vi "read_data_package.vi"(8 "error in (no error)":errorcluster, 11 "OXY_SCPI Reseource In":refnum<visa-resource-name>) -> (0 "error out":errorcluster, 1 "Complete Raw data":string, 2 "Package without Header":string, 3 "OXY_SCPI Reseource Out":refnum<visa-resource-name>)   [LabVIEW 2020, in "OXYGEN_Datastream.lvlib"]
uses:
  OXYGEN_Datastream.lvlib
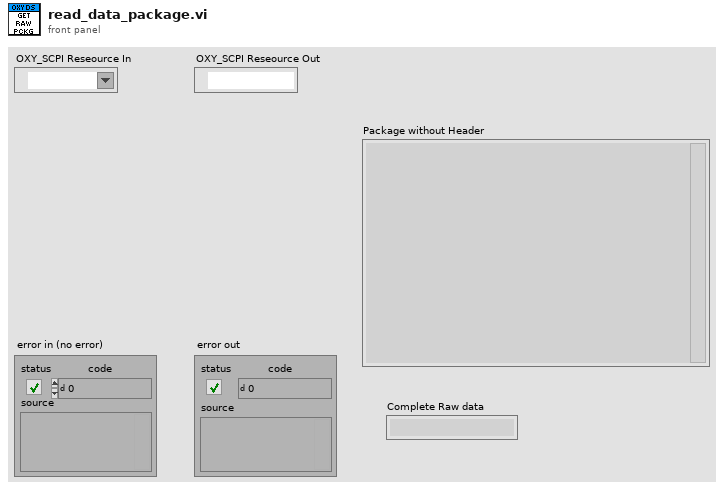
[diagram p1: front panel]
types:
  T1 = enum16{"big-endian, network order", "native, host order", "little-endian"}
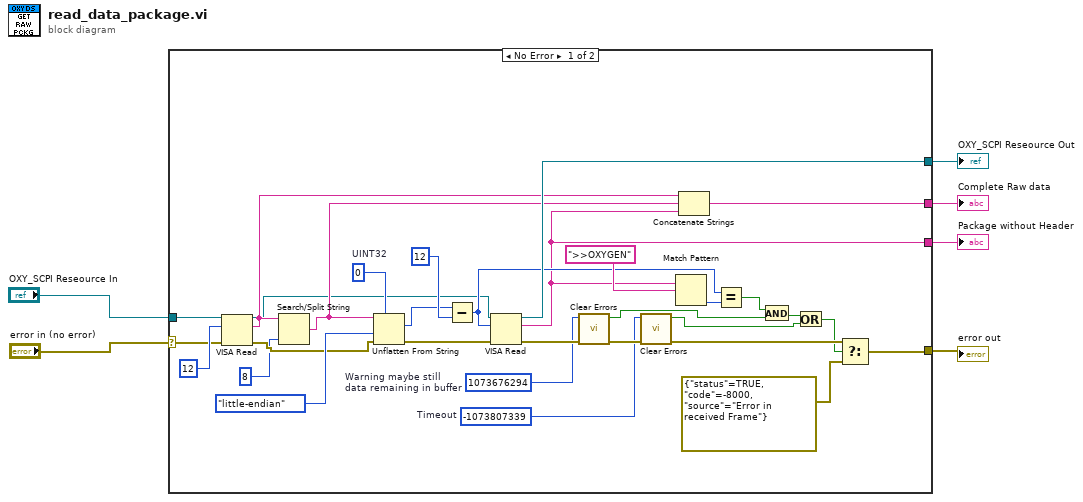
[diagram p0: block diagram]
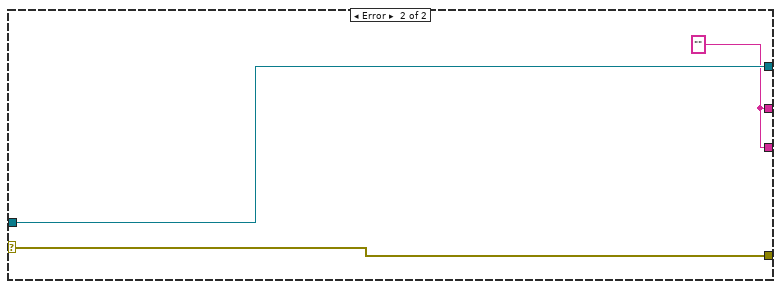
[diagram p2: hidden frame]
diagram:
  n1 = case shown="No Error" "error in (no error)" {
    selector: "error in (no error)" -> [w23 w40]
    tunnel: "OXY_SCPI Reseource In" -> [w31 w39]
    tunnel: [w24 w40] -> w4
    tunnel: [w27 w38] -> w3
    tunnel: [w30 w39] -> w2
    tunnel: [w26 w38] -> w1
    frame No Error {
      w16 = -1073807339  # Timeout
      w17 = 1073676294  # Warning maybe still  data remaining in buffer
      w34 = u32 0  # UINT32
      n2 = VISA Read(VISA resource name=w31, byte count=u32 12, error in (no error)=w23) -> (VISA resource name out=w7:refnum<visa-resource-name>, read buffer=w9:string, error out=w11:errorcluster)  [unwired: 1 out]
      n3 = Search/Split String(string=w9, offset (0)=u32 8 ("byte count")) -> (match + rest of string=w10:string)  [unwired: 1 in, 2 out]
      n4 = Unflatten From String(type=w34, binary string=w10, byte order (0:big-endian, network order)=T1."little-endian", error in (no error)=w11) -> (value=w22:u32, error out=w25:errorcluster)  [unwired: 1 in, 1 out]
      n5 = Subtract(x=w22, y=u32 12) -> (x-y=w28:u32)
      n6 = VISA Read(VISA resource name=w7, byte count=w28, error in (no error)=w25) -> (VISA resource name out=w30:refnum<visa-resource-name>, read buffer=w27:string, error out=w21:errorcluster)  [unwired: 1 out]
      n7 = call <vilib>:"Clear Errors.vi"("error in (no error)"=w21, "specific error code to clear (0: all)"=w17) -> ("error out"=w19:errorcluster, "specific error cleared?"=w15:bool)  [unwired: 4 in]
      n8 = call <vilib>:"Clear Errors.vi"("error in (no error)"=w19, "specific error code to clear (0: all)"=w16) -> ("error out"=w18:errorcluster, "specific error cleared?"=w13:bool)  [unwired: 4 in]
      n9 = Match Pattern(string=w27, regular expression=">>OXYGEN") -> (offset past match=w32:i32)  [unwired: 1 in, 3 out]
      n10 = Concatenate Strings(w9, w10, w27) -> (w26:string)
      n11 = Equal?(x=w28, y=w32) -> (x = y?=w20:bool)
      n12 = And(x=w20, y=w15) -> (x .and. y?=w14:bool)
      n13 = Or(x=w14, y=w13) -> (x .or. y?=w12:bool)
      n14 = Select(t=w18, s=w12, f=errorcluster {"status"=TRUE, "code"=-8000, "source"="Error in received Frame"} ("error IO")) -> (s? t:f=w24:errorcluster)
    }
    frame Error {
      w38 = "" ("read buffer")
    }
  }
  "error out" <- w4
  "Package without Header" <- w3
  "OXY_SCPI Reseource Out" <- w2
  "Complete Raw data" <- w1
